vi "Post-Uninstall Custom Action.vi"(10 "Variant":variant) -> (0 "error out":errorcluster)   [LabVIEW 2020]
uses:
  <vilib>/zip/NI_Unzip.lvlib
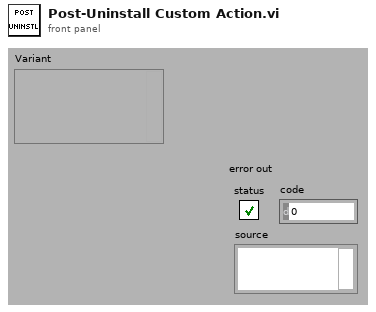
[diagram p1: front panel]
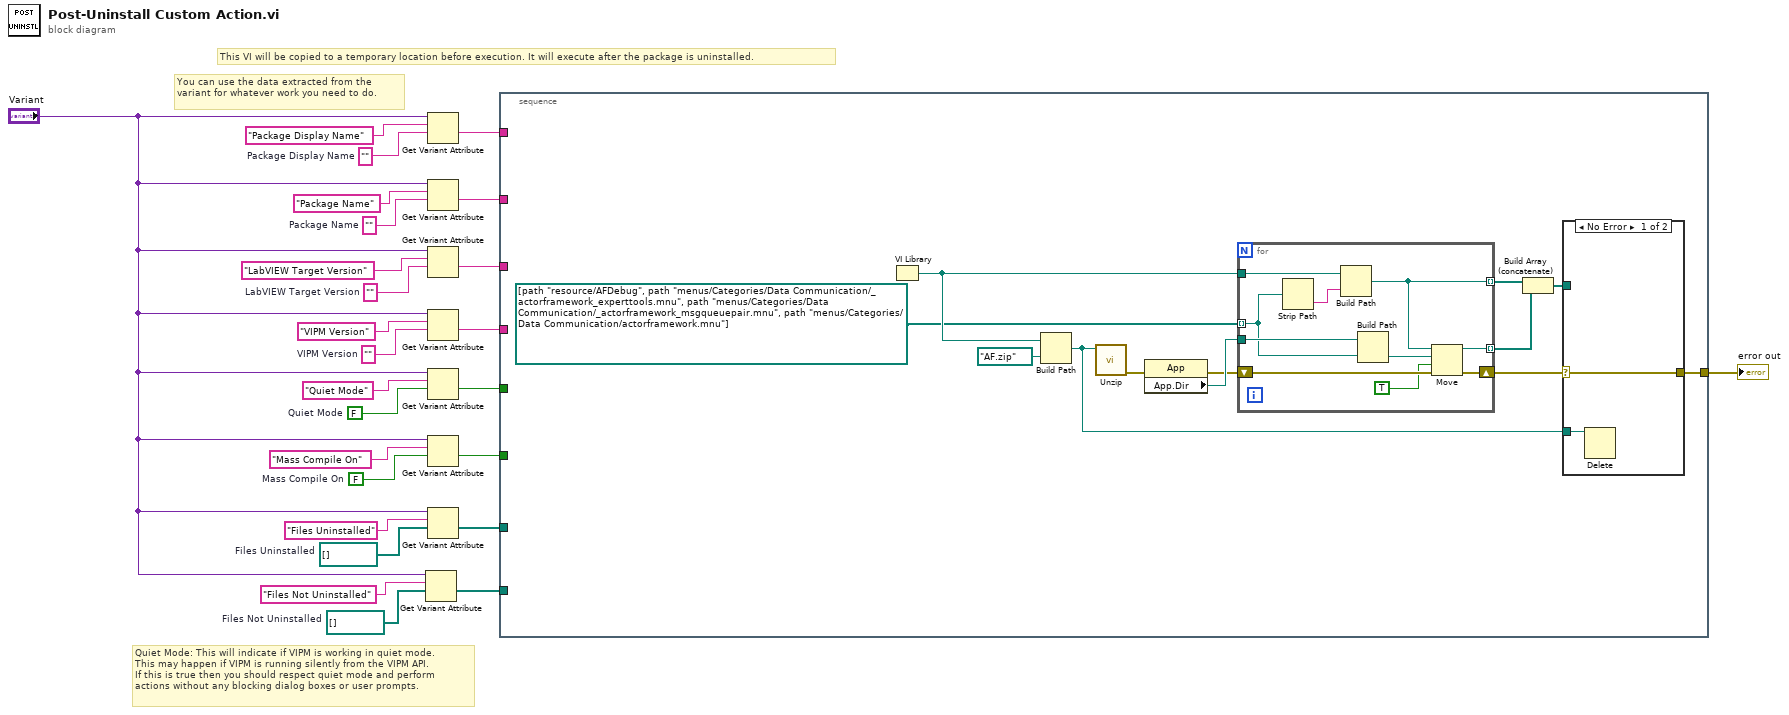
[diagram p0: block diagram]
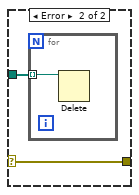
[diagram p2: hidden frame]
diagram:
  w2 = path[] []  # Files Not Uninstalled
  w3 = path[] []  # Files Uninstalled
  w9 = FALSE  # Mass Compile On
  w10 = ""  # Package Display Name
  w17 = FALSE  # Quiet Mode
  w20 = ""  # VIPM Version
  w22 = ""  # LabVIEW Target Version
  w24 = ""  # Package Name
  # "You can use the data extracted from the variant for whatever work you need to do."
  # "Quiet Mode: This will indicate if VIPM is working in quiet mode.\nThis may happen if VIPM is running silently from the VIPM API.\nIf this is true then you should respect quiet mode and perform\nactions without any blocking dialog boxes or user prompts."
  # "This VI will be copied to a temporary location before execution. It will execute after the package is uninstalled."
  n1 = Get Variant Attribute(Variant="Variant", name="Files Not Uninstalled", default value (empty Variant)=w2) -> (value=w7:path[])  [unwired: 1 in, 3 out]
  n2 = Get Variant Attribute(Variant="Variant", name="Package Display Name", default value (empty Variant)=w10) -> (value=w16:string)  [unwired: 1 in, 3 out]
  n3 = Get Variant Attribute(Variant="Variant", name="Package Name", default value (empty Variant)=w24) -> (value=w15:string)  [unwired: 1 in, 3 out]
  n4 = Get Variant Attribute(Variant="Variant", name="LabVIEW Target Version", default value (empty Variant)=w22) -> (value=w14:string)  [unwired: 1 in, 3 out]
  n5 = Get Variant Attribute(Variant="Variant", name="VIPM Version", default value (empty Variant)=w20) -> (value=w13:string)  [unwired: 1 in, 3 out]
  n6 = Get Variant Attribute(Variant="Variant", name="Quiet Mode", default value (empty Variant)=w17) -> (value=w12:bool)  [unwired: 1 in, 3 out]
  n7 = Get Variant Attribute(Variant="Variant", name="Mass Compile On", default value (empty Variant)=w9) -> (value=w11:bool)  [unwired: 1 in, 3 out]
  n8 = Get Variant Attribute(Variant="Variant", name="Files Uninstalled", default value (empty Variant)=w3) -> (value=w6:path[])  [unwired: 1 in, 3 out]
  n9 = stacked-sequence {
    tunnel: w16 -> [_]
    tunnel: w15 -> [_]
    tunnel: w14 -> [_]
    tunnel: w13 -> [_]
    tunnel: w12 -> [_]
    tunnel: w11 -> [_]
    tunnel: w6 -> [_]
    tunnel: w7 -> [_]
    tunnel: [w38] -> w1
    frame #0 {
      n10 = VI Library() -> (path=w31:path)
      n11 = Build Path(base path=w31, name or relative path=path "AF.zip") -> (appended path=w37:path)
      n12 = call <vilib>:"Unzip.vi"("Zip file"=w37) -> ("error out"=w29:errorcluster)  [unwired: 8 in, 2 out]
      n13 = property class="App"(error in=w29) -> (error out=w30:errorcluster, "App.Dir"=w32:path)  [unwired: 1 in, 1 out]
      n14 = for {
        tunnel: w31 -> [w52]
        shift-right: [w51] -> w36
        shift-left: w30 -> [w53]
        tunnel: path[] [path "resource/AFDebug", path "menus/Categories/Data Communication/_actorframework_experttools.mnu", path "menus/Categories/Data Communication/_actorframework_msgqueuepair.mnu", path "menus/Categories/Data Communication/actorframework.mnu"] -> [w48] mode=indexing
        tunnel: w32 -> [w49]
        tunnel: [w45] -> w33 mode=indexing
        tunnel: [w44] -> w35 mode=indexing
        n15 = Strip Path(path=w48) -> (name=w47:string)  [unwired: 1 out]
        n16 = Build Path(base path=w52, name or relative path=w47) -> (appended path=w45:path)
        n17 = Build Path(base path=w49, name or relative path=w48) -> (appended path=w50:path)
        n18 = Move(source path=w45, error in=w53, 9:TRUE ("overwrite (F)"), 10:w50) -> (error out=w51:errorcluster, 3:w44:path)  [unwired: 1 in, 1 out]
      }
      n19 = Build Array (concatenate)(w33, w35) -> (w34:path[])
      n20 = case shown="No Error" w36 {
        selector: w36 -> [w39 w41]
        tunnel: w34 -> [_ w42]
        tunnel: [w39 w41] -> w38
        tunnel: w37 -> [w40 _]
        frame No Error {
          n21 = Delete(path (use dialog)=w40) -> ()  [unwired: 4 in, 3 out]
        }
        frame Error {
          n22 = for {
            tunnel: w42 -> [w43] mode=indexing
            n23 = Delete(path (use dialog)=w43) -> ()  [unwired: 4 in, 3 out]
          }
        }
      }
    }
  }
  "error out" <- w1
